vi "BinaryPlot.vi"() -> ()   [LabVIEW 2010]
panel:
  in  "Plot Legend":i32(listbox)
  in  "AutoScale":bool
  in  "Select All":bool
  out "Waveform Chart":sgl[][](graph)
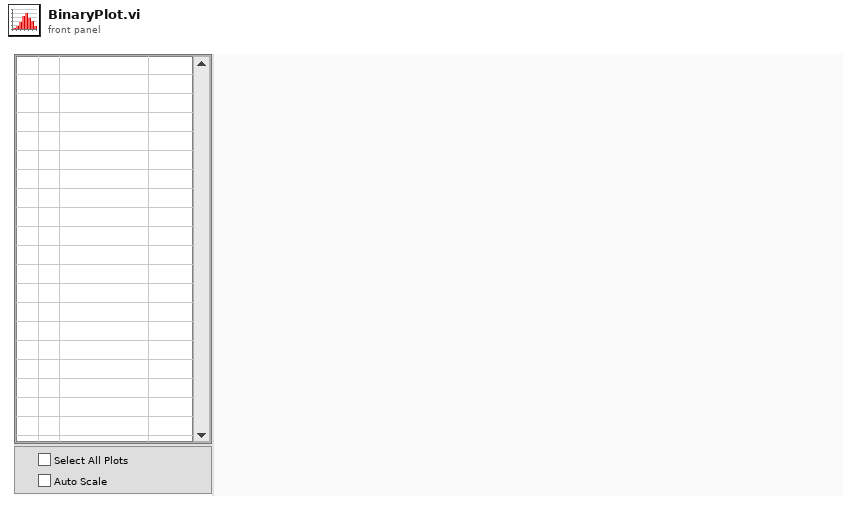
[diagram p1: front panel]
types:
  T1 = cluster{"Error":errorcluster, "PlotNames":string[], "GUIQueue":refnum<queue>, "Telemetry":string, "Format":string, "Buffer":u8[], "BufferIndex":i32, "DataSize":i32, "SearchIndex":i32}
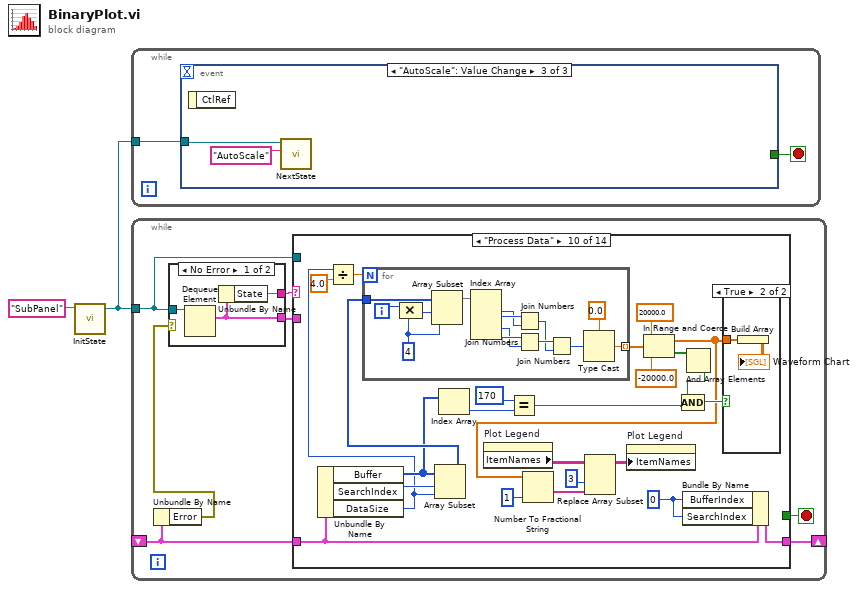
[diagram p0: block diagram]
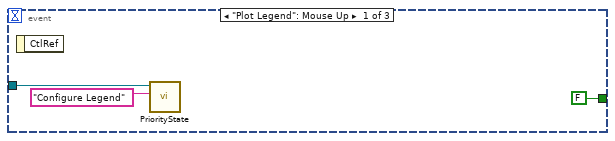
[diagram p2: hidden frame]
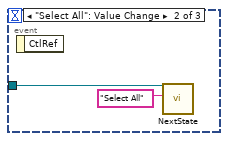
[diagram p3: hidden frame]
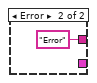
[diagram p4: hidden frame]
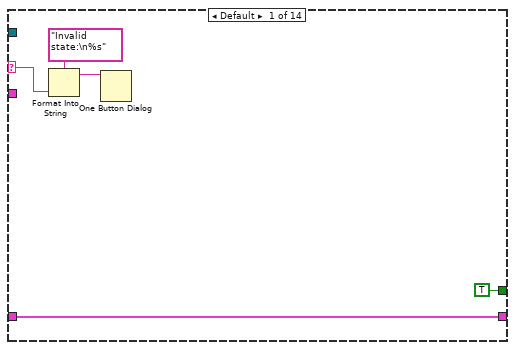
[diagram p5: hidden frame]
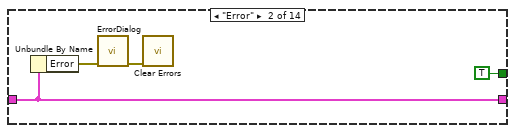
[diagram p6: hidden frame]
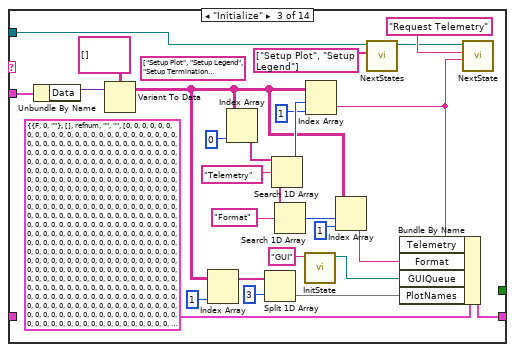
[diagram p7: hidden frame]
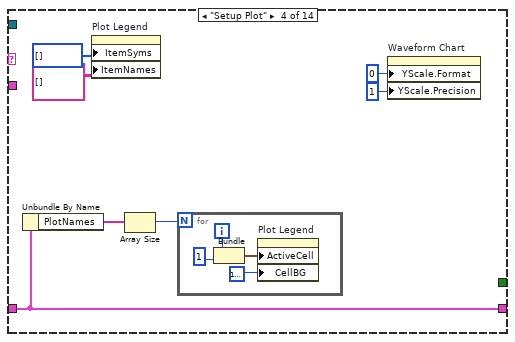
[diagram p8: hidden frame]
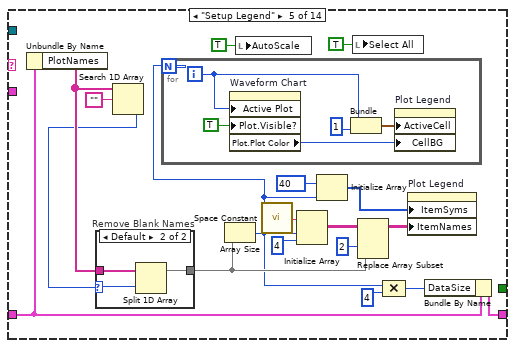
[diagram p9: hidden frame]
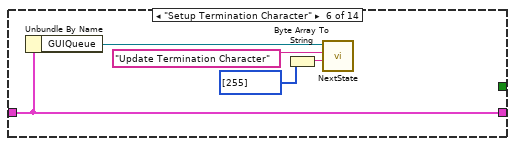
[diagram p11: hidden frame]
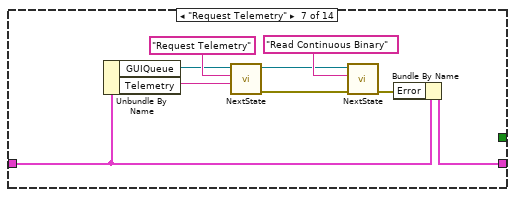
[diagram p12: hidden frame]
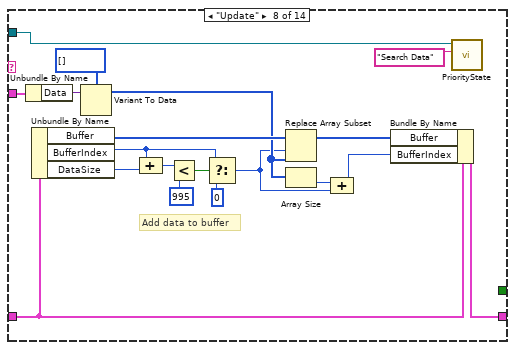
[diagram p13: hidden frame]
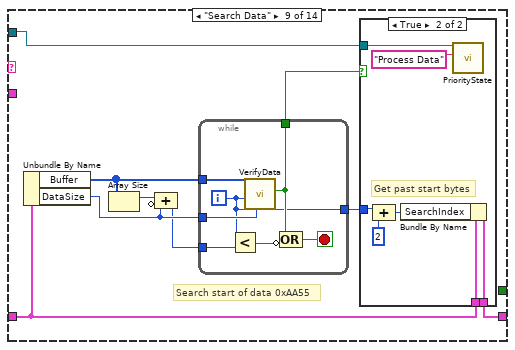
[diagram p14: hidden frame]
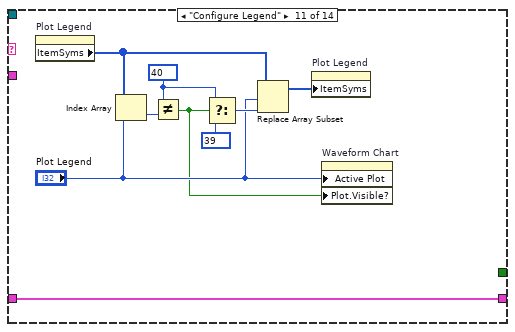
[diagram p17: hidden frame]
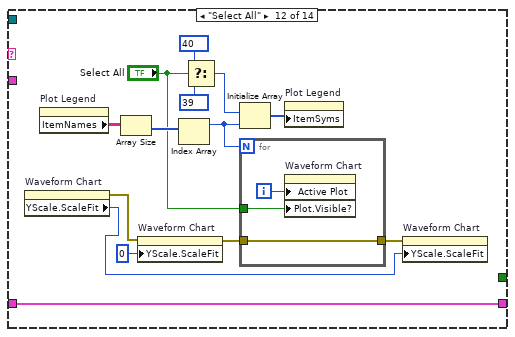
[diagram p18: hidden frame]
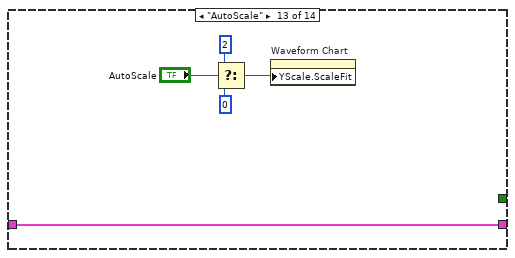
[diagram p19: hidden frame]
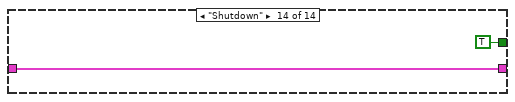
[diagram p20: hidden frame]
diagram:
  n1 = call "InitState.vi"("Name"="SubPanel" ("name (unnamed)")) -> ("Queue Out"=w1:refnum<queue>)  [unwired: 8 in, 1 out]
  n2 = while {
    tunnel: w1 -> [w3]
    stop <- w4 stop-if-true
    n3 = event shown="[2] \"AutoScale\": Value Change" {
      selector: _ -> [_ _ _]
      dyn-events: _ -> [_ _ _]
      timeout: _ -> [_ _ _]
      tunnel: [FALSE _ _] -> w4
      tunnel: w3 -> [w6 w9 w10]
      event "Plot Legend": Mouse Up {
        n4 = event-data() -> ()  [unwired: 1 in, 1 out]
        n5 = call "PriorityState.vi"("State"="Configure Legend", "Queue In"=w6) -> ()  [unwired: 8 in, 2 out]
      }
      event "Select All": Value Change {
        n6 = event-data() -> ()  [unwired: 1 in, 1 out]
        n7 = call "NextState.vi"("State"="Select All", "Queue In"=w9) -> ()  [unwired: 8 in, 2 out]
      }
      event "AutoScale": Value Change {
        n8 = event-data() -> ()  [unwired: 1 in, 1 out]
        n9 = call "NextState.vi"("State"="AutoScale", "Queue In"=w10) -> ()  [unwired: 8 in, 2 out]
      }
    }
  }
  n10 = while {
    tunnel: w1 -> [w12]
    shift-right: [w18] -> _
    shift-left: _ -> [w17]
    stop <- w16 stop-if-true
    n11 = Unbundle By Name(w17) -> ("Error"=w15:errorcluster)
    n12 = case shown="No Error" w15 {
      tunnel: [w21 "Error" ("State")] -> w14
      tunnel: [w20 _] -> w13
      tunnel: w12 -> [w19 _]
      frame No Error {
        n13 = Dequeue Element(queue=w19) -> (element=w20:cluster{"State":string, "Data":variant})  [unwired: 2 in, 3 out]
        n14 = Unbundle By Name(w20) -> ("State"=w21:string)
      }
      frame Error {
      }
    }
    n15 = case shown="\"Process Data\"" w14 {
      selector: w14 -> [w25 _ _ _ _ _ _ _ _ _ _ _ _ _]
      tunnel: w13 -> [_ _ w36 _ _ _ _ w128 _ _ _ _ _ _]
      tunnel: w12 -> [_ _ w33 _ _ _ _ w113 w137 _ _ _ _ _]
      tunnel: [w24 w30 w55 w58 w72 w100 w106 w122 w135 w174 w201 w209 w221 w225] -> w18
      tunnel: w17 -> [w24 w30 _ w58 w73 w100 w108 w123 w136 w175 w201 w209 w221 w225]
      tunnel: [TRUE TRUE _ _ _ _ _ _ _ _ _ _ _ TRUE] -> w16
      frame Default {
        n16 = Format Into String(format string="Invalid state:\n%s", w25) -> (resulting string=w26:string)  [unwired: 2 in, 1 out]
        n17 = One Button Dialog(message=w26) -> ()  [unwired: 1 in, 1 out]
      }
      frame "Error" {
        n18 = Unbundle By Name(w30) -> ("Error"=w29:errorcluster)
        n19 = call "ErrorDialog.vi"("error in"=w29) -> ("error out"=w28:errorcluster)  [unwired: 10 in]
        n20 = call <vilib>:"Clear Errors.vi"("error in (no error)"=w28) -> ()  [unwired: 6 in, 1 out]
      }
      frame "Initialize" {
        (unwired) string[] ["Setup Plot", "Setup Legend", "Setup Termination Character"]
        n21 = Unbundle By Name(w36) -> ("Data"=w35:variant)
        n22 = Variant To Data(Variant=w35, type=string[][] [] ("subarray")) -> (data=w39:string[][])  [unwired: 1 in, 1 out]
        n23 = Index Array(array=w39, index (col)=1 ("disabled index (col)")) -> (element=w53:string[])  [unwired: 1 in]
        n24 = Index Array(array=w39, index (col)=0 ("index (row)")) -> (element=w43:string[])  [unwired: 1 in]
        n25 = Split 1D Array(array=w53, index=3) -> (second subarray=w51:string[])  [unwired: 1 out]
        n26 = Search 1D Array(1D array=w43, element="Telemetry") -> (index of element=w45:i32)  [unwired: 1 in]
        n27 = Search 1D Array(1D array=w43, element="Format") -> (index of element=w40:i32)  [unwired: 1 in]
        n28 = call "InitState.vi"("Name"="GUI") -> ("Queue Out"=w49:refnum<queue>)  [unwired: 8 in, 1 out]
        n29 = Index Array(array=w39, index (row)=w45, index (col)=1 ("index (row)")) -> (element=w37:string)
        n30 = Index Array(array=w39, index (row)=w40, index (col)=1 ("disabled index (col)")) -> (element=w38:string)
        n31 = call "NextStates.vi"("States"=string[] ["Setup Plot", "Setup Legend"], "Queue In"=w33) -> ("Queue Out"=w34:refnum<queue>)  [unwired: 8 in, 1 out]
        n32 = Bundle By Name(cluster=T1 {"Error"={"status"=FALSE, "code"=0, "source"=""}, "PlotNames"=[], "GUIQueue"=refnum, "Telemetry"="", "Format"="", "Buffer"=[0, 0, 0, 0, 0, 0, 0, 0, 0, 0, 0, 0, 0, 0, 0, 0, 0, 0, 0, 0, 0, 0, 0, 0, 0, 0, 0, 0, 0, 0, 0, 0, 0, 0, 0, 0, 0, 0, 0, 0, 0, 0, 0, 0, 0, 0, 0, 0, 0, 0, 0, 0, 0, 0, 0, 0, 0, 0, 0, 0, 0, 0, 0, 0, 0, 0, 0, 0, 0, 0, 0, 0, 0, 0, 0, 0, 0, 0, 0, 0, 0, 0, 0, 0, 0, 0, 0, 0, 0, 0, 0, 0, 0, 0, 0, 0, 0, 0, 0, 0, 0, 0, 0, 0, 0, 0, 0, 0, 0, 0, 0, 0, 0, 0, 0, 0, 0, 0, 0, 0, 0, 0, 0, 0, 0, 0, 0, 0, 0, 0, 0, 0, 0, 0, 0, 0, 0, 0, 0, 0, 0, 0, 0, 0, 0, 0, 0, 0, 0, 0, 0, 0, 0, 0, 0, 0, 0, 0, 0, 0, 0, 0, 0, 0, 0, 0, 0, 0, 0, 0, 0, 0, 0, 0, 0, 0, 0, 0, 0, 0, 0, 0, 0, 0, 0, 0, 0, 0, 0, 0, 0, 0, 0, 0, 0, 0, 0, 0, 0, 0, 0, 0, 0, 0, 0, 0, 0, 0, 0, 0, 0, 0, 0, 0, 0, 0, 0, 0, 0, 0, 0, 0, 0, 0, 0, 0, 0, 0, 0, 0, 0, 0, 0, 0, 0, 0, 0, 0, 0, 0, 0, 0, 0, 0, 0, 0, 0, 0, 0, 0, 0, 0, 0, 0, 0, 0, 0, 0, 0, 0, 0, 0, 0, 0, 0, 0, 0, 0, 0, 0, 0, 0, 0, 0, 0, 0, 0, 0, 0, 0, 0, 0, 0, 0, 0, 0, 0, 0, 0, 0, 0, 0, 0, 0, 0, 0, 0, 0, 0, 0, 0, 0, 0, 0, 0, 0, 0, 0, 0, 0, 0, 0, 0, 0, 0, 0, 0, 0, 0, 0, 0, 0, 0, 0, 0, 0, 0, 0, 0, 0, 0, 0, 0, 0, 0, 0, 0, 0, 0, 0, 0, 0, 0, 0, 0, 0, 0, 0, 0, 0, 0, 0, 0, 0, 0, 0, 0, 0, 0, 0, 0, 0, 0, 0, 0, 0, 0, 0, 0, 0, 0, 0, 0, 0, 0, 0, 0, 0, 0, 0, 0, 0, 0, 0, 0, 0, 0, 0, 0, 0, 0, 0, 0, 0, 0, 0, 0, 0, 0, 0, 0, 0, 0, 0, 0, 0, 0, 0, 0, 0, 0, 0, 0, 0, 0, 0, 0, 0, 0, 0, 0, 0, 0, 0, 0, 0, 0, 0, 0, 0, 0, 0, 0, 0, 0, 0, 0, 0, 0, 0, 0, 0, 0, 0, 0, 0, 0, 0, 0, 0, 0, 0, 0, 0, 0, 0, 0, 0, 0, 0, 0, 0, 0, 0, 0, 0, 0, 0, 0, 0, 0, 0, 0, 0, 0, 0, 0, 0, 0, 0, 0, 0, 0, 0, 0, 0, 0, 0, 0, 0, 0, 0, 0, 0, 0, 0, 0, 0, 0, 0, 0, 0, 0, 0, 0, 0, 0, 0, 0, 0, 0, 0, 0, 0, 0, 0, 0, 0, 0, 0, 0, 0, 0, 0, 0, 0, 0, 0, 0, 0, 0, 0, 0, 0, 0, 0, 0, 0, 0, 0, 0, 0, 0, 0, 0, 0, 0, 0, 0, 0, 0, 0, 0, 0, 0, 0, 0, 0, 0, 0, 0, 0, 0, 0, 0, 0, 0, 0, 0, 0, 0, 0, 0, 0, 0, 0, 0, 0, 0, 0, 0, 0, 0, 0, 0, 0, 0, 0, 0, 0, 0, 0, 0, 0, 0, 0, 0, 0, 0, 0, 0, 0, 0, 0, 0, 0, 0, 0, 0, 0, 0, 0, 0, 0, 0, 0, 0, 0, 0, 0, 0, 0, 0, 0, 0, 0, 0, 0, 0, 0, 0, 0, 0, 0, 0, 0, 0, 0, 0, 0, 0, 0, 0, 0, 0, 0, 0, 0, 0, 0, 0, 0, 0, 0, 0, 0, 0, 0, 0, 0, 0, 0, 0, 0, 0, 0, 0, 0, 0, 0, 0, 0, 0, 0, 0, 0, 0, 0, 0, 0, 0, 0, 0, 0, 0, 0, 0, 0, 0, 0, 0, 0, 0, 0, 0, 0, 0, 0, 0, 0, 0, 0, 0, 0, 0, 0, 0, 0, 0, 0, 0, 0, 0, 0, 0, 0, 0, 0, 0, 0, 0, 0, 0, 0, 0, 0, 0, 0, 0, 0, 0, 0, 0, 0, 0, 0, 0, 0, 0, 0, 0, 0, 0, 0, 0, 0, 0, 0, 0, 0, 0, 0, 0, 0, 0, 0, 0, 0, 0, 0, 0, 0, 0, 0, 0, 0, 0, 0, 0, 0, 0, 0, 0, 0, 0, 0, 0, 0, 0, 0, 0, 0, 0, 0, 0, 0, 0, 0, 0, 0, 0, 0, 0, 0, 0, 0, 0, 0, 0, 0, 0, 0, 0, 0, 0, 0, 0, 0, 0, 0, 0, 0, 0, 0, 0, 0, 0, 0, 0, 0, 0, 0, 0, 0, 0, 0, 0, 0, 0, 0, 0, 0, 0, 0, 0, 0, 0, 0, 0, 0, 0, 0, 0, 0, 0, 0, 0, 0, 0, 0, 0, 0, 0, 0, 0, 0, 0, 0, 0, 0, 0, 0, 0, 0, 0, 0, 0, 0, 0, 0, 0, 0, 0, 0, 0, 0, 0, 0, 0, 0, 0, 0, 0, 0, 0, 0, 0, 0, 0, 0, 0, 0, 0, 0, 0, 0, 0, 0, 0, 0, 0, 0, 0, 0, 0, 0, 0, 0, 0, 0, 0, 0, 0, 0, 0, 0, 0, 0, 0, 0, 0, 0, 0, 0, 0, 0, 0, 0, 0, 0, 0, 0, 0, 0, 0, 0, 0, 0, 0, 0, 0, 0, 0, 0, 0, 0, 0, 0, 0, 0, 0, 0, 0, 0, 0, 0, 0, 0, 0, 0, 0, 0, 0, 0, 0, 0, 0, 0, 0, 0, 0, 0, 0, 0, 0, 0, 0, 0, 0, 0, 0, 0, 0, 0, 0, 0, 0, 0, 0, 0, 0, 0, 0, 0, 0, 0, 0, 0, 0, 0], "BufferIndex"=0, "DataSize"=48, "SearchIndex"=0}, "Telemetry"=w37, "Format"=w38, "GUIQueue"=w49, "PlotNames"=w51) -> (w55:T1)
        n33 = call "NextState.vi"("Data"=w37, "State"="Request Telemetry", "Queue In"=w34) -> ()  [unwired: 7 in, 2 out]
      }
      frame "Setup Plot" {
        n34 = Unbundle By Name(w58) -> ("PlotNames"=w60:string[])
        n35 = property on="Plot Legend" class="MCListbox (strict)"("ItemSyms"=i32[] [] ("Item Symbols"), "ItemNames"=string[][] [] ("Item Names")) -> ()  [unwired: 2 in, 2 out]
        n36 = Array Size(array=w60) -> (size(s)=w59:i32)
        n37 = for {
          N: w59 -> [_]
          i -> [w66]
          n38 = Bundle(w66, 1) -> (w68:cluster{i32, i32})  [unwired: 1 in]
          n39 = property on="Plot Legend" class="MCListbox (strict)"("ActiveCell"=w68, "CellBG"=u32 16777216) -> ()  [unwired: 2 in, 2 out]
        }
        n40 = property on="Waveform Chart" class="WFChart (strict)"("YScale.Format"=u8 0 ("Y Scale.Display Format:Format"), "YScale.Precision"=u8 1 ("Y Scale.Display Format:Precision")) -> ()  [unwired: 2 in, 2 out]
      }
      frame "Setup Legend" {
        n41 = Unbundle By Name(w73) -> ("PlotNames"=w78:string[])
        n42 = Search 1D Array(1D array=w78, element="") -> (index of element=w76:i32)  [unwired: 1 in]
        n43 = case "Remove Blank Names" shown="Default" w76 {
          selector: w76 -> [_ w88]
          tunnel: w78 -> [w87 w90]
          tunnel: [w87 w89] -> w77
          frame -1 {
          }
          frame Default {
            n44 = Split 1D Array(array=w90, index=w88) -> (first subarray=w89:string[])  [unwired: 1 out]
          }
        }
        n45 = Array Size(array=w77) -> (size(s)=w71:i32)
        n46 = for {
          N: w71 -> [_]
          i -> [w92]
          n47 = property on="Waveform Chart" class="WFChart (strict)"("Active Plot"=w92, "Plot.Visible?"=TRUE ("Plot.Visible")) -> ("Plot.Plot Color"=w91:u32)  [unwired: 2 in, 2 out]
          n48 = Bundle(w92, 1) -> (w94:cluster{i32, i32})  [unwired: 1 in]
          n49 = property on="Plot Legend" class="MCListbox (strict)"("ActiveCell"=w94, "CellBG"=w91) -> ()  [unwired: 2 in, 2 out]
        }
        n50 = local write "AutoScale"(TRUE ("AutoScale")) -> ()
        n51 = call <vilib>:"Space Constant.vi"() -> ("String"=w86:string)
        n52 = Initialize Array(w86, w71, 4 ("dimension size")) -> (w85:string[][])
        n53 = Initialize Array(40, w71) -> (w80:i32[])
        n54 = local write "Select All"(TRUE ("Select All")) -> ()
        n55 = Replace Array Subset(array=w85, new element=w77, index (col)=2 ("disabled index (col)")) -> (w82:string[][])  [unwired: 1 in]
        n56 = Compound Arithmetic op=MULTIPLY(w71, 4 ("value")) -> (w69:i32)
        n57 = property on="Plot Legend" class="MCListbox (strict)"("ItemSyms"=w80, "ItemNames"=w82) -> ()  [unwired: 2 in, 2 out]
        n58 = Bundle By Name(cluster=w73, "DataSize"=w69) -> (w72:T1)
      }
      frame "Setup Termination Character" {
        n59 = Unbundle By Name(w100) -> ("GUIQueue"=w99:refnum<queue>)
        n60 = Byte Array To String(unsigned byte array=u8[] [255]) -> (string=w97:string)
        n61 = call "NextState.vi"("Data"=w97, "State"="Update Termination Character", "Queue In"=w99) -> ()  [unwired: 7 in, 2 out]
      }
      frame "Request Telemetry" {
        n62 = Unbundle By Name(w108) -> ("GUIQueue"=w104:refnum<queue>, "Telemetry"=w103:string)
        n63 = call "NextState.vi"("Data"=w103, "State"="Request Telemetry", "Queue In"=w104) -> ("Error Out"=w101:errorcluster, "Queue Out"=w102:refnum<queue>)  [unwired: 7 in]
        n64 = call "NextState.vi"("Error In"=w101, "State"="Read Continuous Binary", "Queue In"=w102) -> ("Error Out"=w107:errorcluster)  [unwired: 7 in, 1 out]
        n65 = Bundle By Name(cluster=w108, "Error"=w107) -> (w106:T1)
      }
      frame "Update" {
        # "Add data to buffer"
        n66 = Unbundle By Name(w128) -> ("Data"=w127:variant)
        n67 = Unbundle By Name(w123) -> ("Buffer"=w125:u8[], "BufferIndex"=w116:i32, "DataSize"=w111:i32)
        n68 = Variant To Data(Variant=w127, type=u8[] [] ("unsigned byte array")) -> (data=w121:u8[])  [unwired: 1 in, 1 out]
        n69 = Compound Arithmetic op=ADD(w116, w111) -> (w119:i32)
        n70 = Less?(x=w119, y=995) -> (x < y?=w117:bool)
        n71 = Select(t=w116, s=w117, f=0) -> (s? t:f=w114:i32)
        n72 = Replace Array Subset(array=w125, new element=w121, index=w114) -> (w120:u8[])
        n73 = Array Size(array=w121) -> (size(s)=w124:i32)
        n74 = Compound Arithmetic op=ADD(w124, w114) -> (w112:i32)
        n75 = Bundle By Name(cluster=w123, "Buffer"=w120, "BufferIndex"=w112) -> (w122:T1)
        n76 = call "PriorityState.vi"("State"="Search Data", "Queue In"=w113) -> ()  [unwired: 8 in, 2 out]
      }
      frame "Search Data" {
        # "Search start of data 0xAA55"
        n77 = Unbundle By Name(w136) -> ("Buffer"=w130:u8[], "DataSize"=w132:i32)
        n78 = Array Size(array=w130) -> (size(s)=w131:i32)
        n79 = Compound Arithmetic op=ADD(w131, invert w132) -> (w129:i32)
        n80 = while {
          tunnel: w130 -> [w144]
          tunnel: w132 -> [w143]
          tunnel: [w138] -> w134
          tunnel: [w140] -> w133
          tunnel: w129 -> [w142]
          i -> [w138]
          stop <- w139 stop-if-true
          n81 = Less?(x=w138, y=w142) -> (x < y?=w141:bool)
          n82 = call "VerifyData.vi"("Data Size"=w143, "Index"=w138, "Data Buffer"=w144) -> ("Found"=w140:bool)  [unwired: 6 in]
          n83 = Compound Arithmetic op=OR(w140, invert w141) -> (w139:bool)
        }
        n84 = case shown="True" w133 {
          tunnel: w137 -> [_ w150]
          tunnel: w136 -> [w145 w152]
          tunnel: [w145 w151] -> w135
          tunnel: w134 -> [_ w148]
          frame False {
          }
          frame True {
            # "Get past start bytes"
            n85 = Compound Arithmetic op=ADD(w148, 2 ("value")) -> (w146:i32)
            n86 = Bundle By Name(cluster=w152, "SearchIndex"=w146) -> (w151:T1)
            n87 = call "PriorityState.vi"("State"="Process Data", "Queue In"=w150) -> ()  [unwired: 8 in, 2 out]
          }
        }
      }
      frame "Process Data" {
        w173 = 0 ("BufferIndex")
        n88 = Unbundle By Name(w175) -> ("Buffer"=w169:u8[], "SearchIndex"=w170:i32, "DataSize"=w166:i32)
        n89 = Divide(x=w166, y=4.0) -> (x/y=w172:dbl)
        n90 = Array Subset(array=w169, index=w170, length=w166) -> (w171:u8[])
        n91 = for {
          N: w172 -> [_]
          tunnel: w171 -> [w192]
          tunnel: [w179] -> w165 mode=indexing
          i -> [w189]
          w190 = 4 ("length")
          n92 = Compound Arithmetic op=MULTIPLY(w189, w190) -> (w191:i32)
          n93 = Array Subset(array=w192, index=w191, length=w190) -> (w188:u8[])
          n94 = Index Array(array=w188) -> (element #1=w184:u8, element #2=w185:u8, element #3=w186:u8, element #4=w187:u8)  [unwired: 4 in]
          n95 = Join Numbers(hi=w185, lo=w184) -> ((hi.lo)=w182:u16)
          n96 = Join Numbers(hi=w187, lo=w186) -> ((hi.lo)=w183:u16)
          n97 = Join Numbers(hi=w183, lo=w182) -> ((hi.lo)=w180:u32)
          n98 = Type Cast(type=sgl 0.0, x=w180) -> (*(type *) &x=w179:sgl)
        }
        n99 = Index Array(array=w169) -> (element=w167:u8)  [unwired: 1 in]
        n100 = property on="Plot Legend" class="MCListbox (strict)"() -> ("ItemNames"=w157:string[][])  [unwired: 2 in, 2 out]
        n101 = Equal?(x=u8 170 ("y"), y=w167) -> (x = y?=w161:bool)
        n102 = In Range and Coerce(upper limit=sgl 20000.0, x=w165, lower limit=sgl -20000.0) -> (coerced(x)=w153:sgl[], In Range?=w162:bool[])
        n103 = Number To Fractional String(number=w153, precision (6)=i16 1) -> (F-format string=w155:string[])  [unwired: 2 in]
        n104 = Replace Array Subset(array=w157, new element=w155, index (col)=3 ("disabled index (col)")) -> (w156:string[][])  [unwired: 1 in]
        n105 = property on="Plot Legend" class="MCListbox (strict)"("ItemNames"=w156) -> ()  [unwired: 2 in, 2 out]
        n106 = And Array Elements(Boolean array=w162) -> (logical AND=w159:bool)
        n107 = Compound Arithmetic op=AND(w159, w161) -> (w160:bool)
        n108 = Bundle By Name(cluster=w175, "BufferIndex"=w173, "SearchIndex"=w173) -> (w174:T1)
        n109 = case shown="True" w160 {
          tunnel: w153 -> [_ w178]
          frame False {
          }
          frame True {
            n110 = Build Array(w178) -> (→"Waveform Chart":sgl[][])
          }
        }
      }
      frame "Configure Legend" {
        w194 = 40
        n111 = property on="Plot Legend" class="MCListbox (strict)"() -> ("ItemSyms"=w199:i32[])  [unwired: 2 in, 2 out]
        n112 = Index Array(array=w199, index="Plot Legend") -> (element=w200:i32)
        n113 = Not Equal?(x=w194, y=w200) -> (x != y?=w193:bool)
        n114 = Select(t=w194, s=w193, f=39) -> (s? t:f=w198:i32)
        n115 = Replace Array Subset(array=w199, new element=w198, index="Plot Legend") -> (w197:i32[])
        n116 = property on="Plot Legend" class="MCListbox (strict)"("ItemSyms"=w197) -> ()  [unwired: 2 in, 2 out]
        n117 = property on="Waveform Chart" class="WFChart (strict)"("Active Plot"="Plot Legend", "Plot.Visible?"=w193) -> ()  [unwired: 2 in, 2 out]
      }
      frame "Select All" {
        n118 = property on="Waveform Chart" class="WFChart (strict)"() -> (error out=w203:errorcluster, "YScale.ScaleFit"=w202:u8)  [unwired: 2 in, 1 out]
        n119 = property on="Plot Legend" class="MCListbox (strict)"() -> ("ItemNames"=w210:string[][])  [unwired: 2 in, 2 out]
        n120 = Array Size(array=w210) -> (size(s)=w215:i32[])
        n121 = property on="Waveform Chart" class="WFChart (strict)"(error in=w203, "YScale.ScaleFit"=u8 0 ("Y Scale.Scale Fit")) -> (error out=w205:errorcluster)  [unwired: 1 in, 1 out]
        n122 = Index Array(array=w215) -> (element=w207:i32)  [unwired: 1 in]
        n123 = Select(t=40, s="Select All", f=39) -> (s? t:f=w212:i32)
        n124 = Initialize Array(w212, w207) -> (w211:i32[])
        n125 = for {
          N: w207 -> [_]
          tunnel: "Select All" -> [w217]
          tunnel: w205 -> [w216]
          tunnel: [w216] -> w204
          i -> [w218]
          n126 = property on="Waveform Chart" class="WFChart (strict)"("Active Plot"=w218, "Plot.Visible?"=w217) -> ()  [unwired: 2 in, 2 out]
        }
        n127 = property on="Plot Legend" class="MCListbox (strict)"("ItemSyms"=w211) -> ()  [unwired: 2 in, 2 out]
        n128 = property on="Waveform Chart" class="WFChart (strict)"(error in=w204, "YScale.ScaleFit"=w202) -> ()  [unwired: 1 in, 2 out]
      }
      frame "AutoScale" {
        n129 = Select(t=u8 2 ("Active Y Scale"), s="AutoScale", f=u8 0 ("Active Y Scale")) -> (s? t:f=w219:u8)
        n130 = property on="Waveform Chart" class="WFChart (strict)"("YScale.ScaleFit"=w219) -> ()  [unwired: 2 in, 2 out]
      }
      frame "Shutdown" {
      }
    }
  }
